vi "Get Project With Two LVUnit Tests.vi"() -> (2 "Project File":path)   [LabVIEW 2017, in "LVUnit Test Discoverer.Tests.lvlib"]
uses:
  LVUnit Test Discoverer.Tests.lvlib
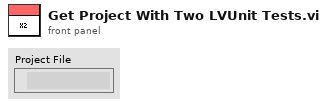
[diagram p1: front panel]
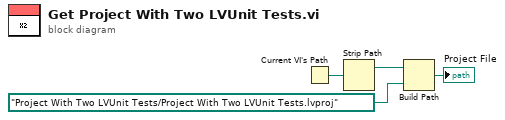
[diagram p0: block diagram]
diagram:
  n1 = Current VI's Path() -> (path=w4:path)
  n2 = Strip Path(path=w4) -> (stripped path=w3:path)  [unwired: 1 out]
  n3 = Build Path(base path=w3, name or relative path=path "Project With Two LVUnit Tests/Project With Two LVUnit Tests.lvproj" ("Path")) -> (appended path=→"Project File":path)
